vi "Set Index.vi"(10 "Index":i32, 11 "Team in":refnum<class "Team.lvclass">) -> (3 "Team out":refnum<class "Team.lvclass">)   [LabVIEW 2020, in "SquareBattle.lvlib" / "Team.lvclass"]
uses:
  Team.lvclass
  Team.lvclass/Team.ctl
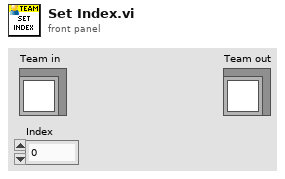
[diagram p1: front panel]
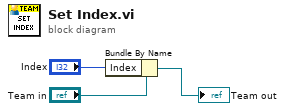
[diagram p0: block diagram]
diagram:
  n1 = Bundle By Name(cluster="Team in", "Index"="Index") -> (→"Team out":refnum<class "Team.lvclass">)
